vi "RVC 2D Coordinate Frames.vi"() -> ()   [LabVIEW 2013]
uses:
  <vilib>/Analysis/Matrix/Datatypes/RealMatrix.ctl
  <vilib>/Analysis/baseanly.llb/Real A x B.vi
  LabVIEW Corke Toolkit/Functions/Position and Orientation/rvc Plot 2D Transform (vector).vi
  <vilib>/Analysis/baseanly.llb/Real Inverse Matrix.vi
  LabVIEW Corke Toolkit/Functions/Position and Orientation/rvc Plot 2D Transform (scalar).vi
  LabVIEW Corke Toolkit/Functions/Position and Orientation/rvc 2D Euler to Homogeneous (vector).vi
  <vilib>/Analysis/NI_AALBase.lvlib
  <vilib>/Analysis/Matrix/NI_Matrix.lvlib
panel:
  out "Homogeneous":T1
  out "P":dbl[](array[numeric])
  out "P":T1
  out "P1":T1
  out "matrix transformation (T4)":picture
  out "matrix transformation (T3)":picture
  out "matrix transformation (T2)":picture
  out "XY Graph":cluster{dbl[], dbl[]}[](graph)
  out "matrix transformation (T1)":picture
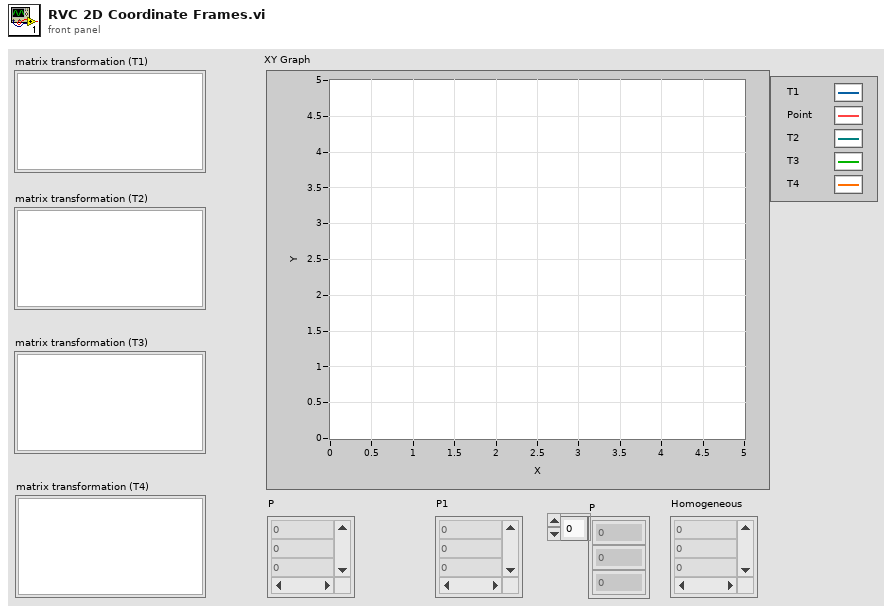
[diagram p1: front panel]
types:
  T1 = typedef "NI_Matrix.lvlib/RealMatrix.ctl" = dbl[][]
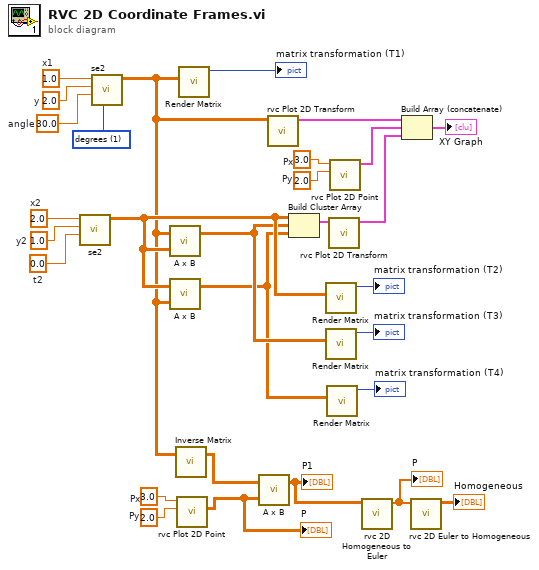
[diagram p0: block diagram]
diagram:
  w7 = 2.0  # Py
  w6 = 3.0  # Px
  w9 = u16 1 items=["radians", "degrees"] ("angle unit")
  w21 = 0.0  # t2
  w20 = 1.0  # y2
  w19 = 2.0  # x2
  w10 = 30.0  # angle
  w28 = 2.0  # y
  w29 = 1.0  # x1
  w22 = 2.0  # Py
  w23 = 3.0  # Px
  n1 = call "se2.vi"("theta"=w21, "y"=w20, "x"=w19) -> ("T"=w15:dbl[][])  [unwired: 7 in, 1 out]
  n2 = call "se2.vi"("angle unit"=w9, "theta"=w10, "y"=w28, "x"=w29) -> ("T"=w8:dbl[][])  [unwired: 6 in, 1 out]
  n3 = call-poly <vilib>:"A x B.vi"("B"=w15, "A"=w8) -> ("A x B"=w13:T1)  [unwired: 1 out]
  n4 = call-poly <vilib>:"A x B.vi"("B"=w8, "A"=w15) -> ("A x B"=w12:T1)  [unwired: 1 out]
  n5 = call-poly <vilib>:"Inverse Matrix.vi"("Input Matrix"=w8) -> ("Inverse Matrix"=w5:T1)  [unwired: 1 in, 1 out]
  n6 = call "rvc Plot 2D Point.vi"("Y"=w7, "X"=w6) -> ("Column vector"=w4:dbl[][])  [unwired: 8 in, 1 out]
  "P" <- w4
  n7 = call "Render Matrix.vi"("A"=w8) -> ("picture out"=→"matrix transformation (T1)":picture)  [unwired: 10 in]
  n8 = call-poly <vilib>:"A x B.vi"("B"=w4, "A"=w5) -> ("A x B"=w3:T1)  [unwired: 1 out]
  "P1" <- w3
  n9 = call-poly "rvc Plot 2D Transform.vi"("T"=w8) -> ("XY Graph 2"=w26:cluster{dbl[], dbl[]})  [unwired: 9 in, 1 out]
  n10 = Build Cluster Array(w15, w13, w12) -> (w18:cluster{"A x B":T1}[])
  n11 = call "Render Matrix.vi"("A"=w15) -> ("picture out"=→"matrix transformation (T2)":picture)  [unwired: 10 in]
  n12 = call "Render Matrix.vi"("A"=w13) -> ("picture out"=→"matrix transformation (T3)":picture)  [unwired: 10 in]
  n13 = call "Render Matrix.vi"("A"=w12) -> ("picture out"=→"matrix transformation (T4)":picture)  [unwired: 10 in]
  n14 = call-poly "rvc Plot 2D Transform.vi"("Array of transformations"=w18) -> ("XY Graph"=w17:cluster{dbl[], dbl[]}[])  [unwired: 9 in, 1 out]
  n15 = call "rvc Plot 2D Point.vi"("Y"=w22, "X"=w23) -> ("XY Graph"=w24:cluster{dbl[], dbl[]})  [unwired: 8 in, 1 out]
  n16 = call "rvc 2D Homogeneous to Euler.vi"("T"=w3) -> ("Array"=w2:dbl[])  [unwired: 7 in, 3 out]
  "P" <- w2
  n17 = Build Array (concatenate)(w26, w24, w17) -> (→"XY Graph":cluster{dbl[], dbl[]}[])
  n18 = call-poly "rvc 2D Euler to Homogeneous.vi"("Euler"=w2) -> ("Homogeneous"=→"Homogeneous":T1)  [unwired: 9 in, 1 out]
